vi "termometr.vi"() -> ()   [LabVIEW 2022 SP3]
panel:
  in  "Numeric":i16
  out "uwaga!!!":bool
  out "uwaga":bool
  in  "Knob":dbl(knob) scale=35.0..44.0
  out "Thermometer":dbl(slide) scale=35.0..44.0
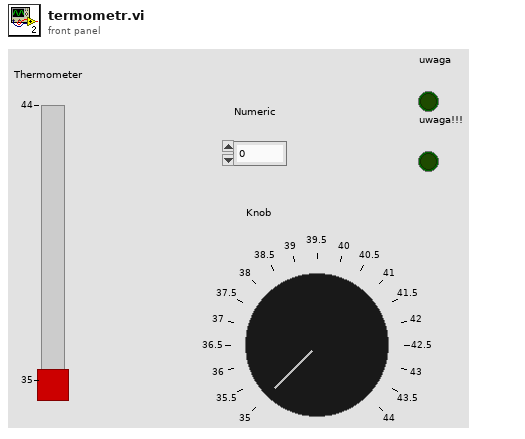
[diagram p1: front panel]
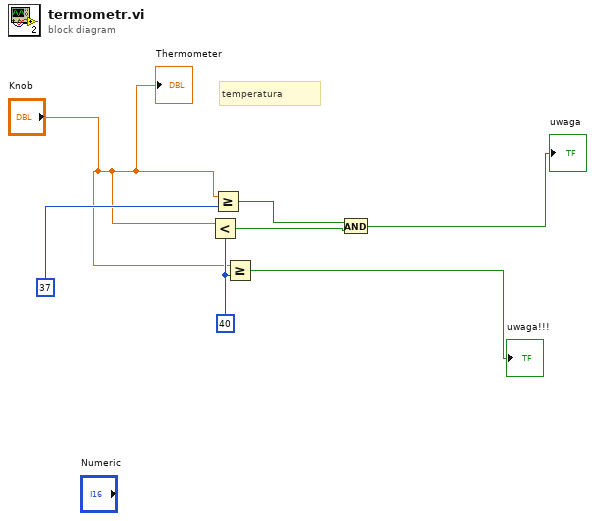
[diagram p0: block diagram]
diagram:
  w4 = 40
  # "temperatura"
  n1 = Less?(x="Knob", y=w4) -> (x < y?=w3:bool)
  n2 = Greater Or Equal?(x="Knob", y=37) -> (x >= y?=w5:bool)
  n3 = Greater Or Equal?(x="Knob", y=w4) -> (x >= y?=→"uwaga!!!":bool)
  n4 = And(x=w5, y=w3) -> (x .and. y?=→"uwaga":bool)
  "Thermometer" <- "Knob"
